vi "WLAN_RSMA_FrameBuild - 2SC.vi"(4 "No. Common Bits":i32=3, 6 "No. Total Bits":i32=6, 7 "Alpha":dbl min=0.0 max=1.0 step=0.05 format="%#_13g", 8 "error in (no error)":errorcluster, 9 "data in 2":i8[](array[numeric]) caption="input bit stream", 10 "Modulation parameter":T1, 11 "data in":i8[](array[numeric]) caption="input bit stream") -> (0 "error out":errorcluster, 3 "output array":cdb[](array[numeric]))   [LabVIEW 2022 SP3]
panel:
  out "Constellation Map":cdb[](graph)
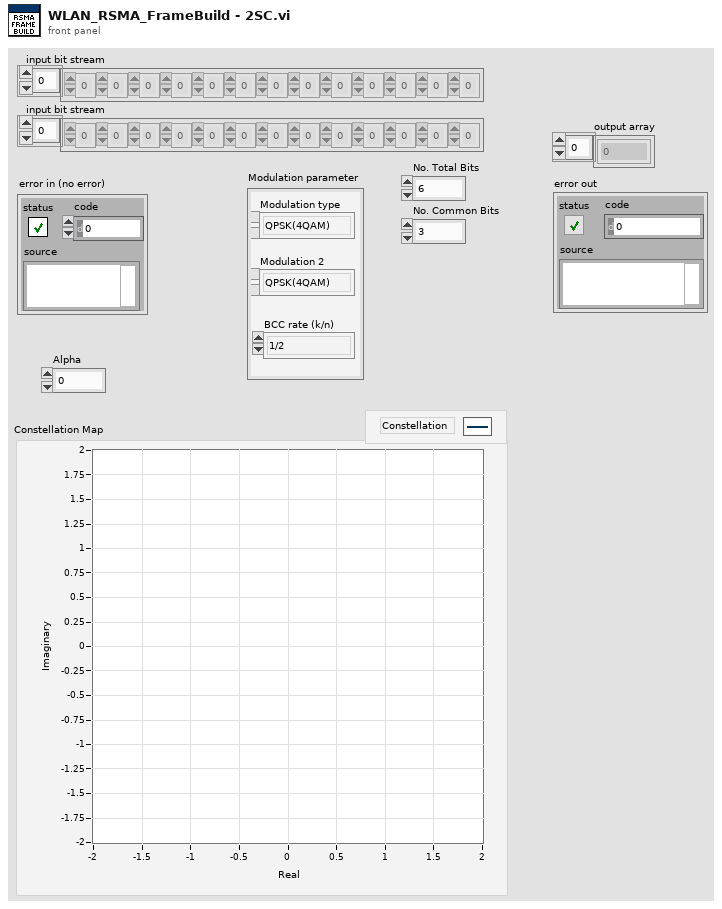
[diagram p1: front panel]
types:
  T1 = cluster{"Modulation type":enum16{"QPSK(4QAM)", "64QAM", "16QAM", "BPSK", "BPSK Vertical"}, "BCC rate (k/n)":enum16{"1/2", "2/3", "3/4"}, "Modulation 2":enum16{"QPSK(4QAM)", "64QAM", "16QAM", "BPSK", "BPSK Vertical"}}
  T2 = enum16{"QPSK(4QAM)", "64QAM", "16QAM", "BPSK", "BPSK Vertical"}
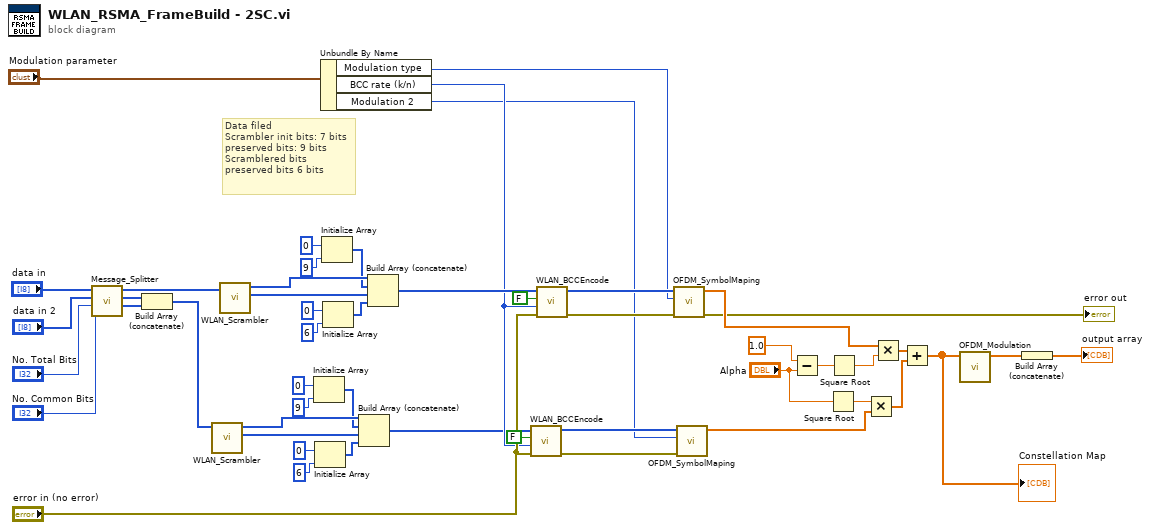
[diagram p0: block diagram]
diagram:
  # "Data filed\nScrambler init bits: 7 bits\npreserved bits: 9 bits\nScramblered bits\npreserved bits 6 bits"
  n1 = call "Message_Splitter.vi"("No. Common Bits"="No. Common Bits", "No. Total Bits"="No. Total Bits", "W2"="data in 2", "W1"="data in") -> ("Wp2"=w9:u8[], "Wp1"=w10:u8[], "Wc"=w8:u8[])  [unwired: 5 in]
  n2 = Build Array (concatenate)(w10, w9) -> (w7:u8[])
  n3 = call "WLAN_Scrambler.vi"("input bit stream"=w7) -> ("scrambled bits"=w27:i8[], "scrambler initial bit"=w31:i8[])  [unwired: 9 in]
  n4 = call "WLAN_Scrambler.vi"("input bit stream"=w8) -> ("scrambled bits"=w23:i8[], "scrambler initial bit"=w38:i8[])  [unwired: 9 in]
  n5 = Initialize Array(i8 0 ("element"), 9 ("dimension size")) -> (w30:i8[])
  n6 = Initialize Array(i8 0 ("element"), 6 ("dimension size")) -> (w24:i8[])
  n7 = Unbundle By Name("Modulation parameter") -> ("Modulation type"=w6:T2, "BCC rate (k/n)"=w46:enum16{"1/2", "2/3", "3/4"}, "Modulation 2"=w3:T2)
  n8 = Initialize Array(i8 0 ("element"), 9 ("dimension size")) -> (w37:i8[])
  n9 = Initialize Array(i8 0 ("element"), 6 ("dimension size")) -> (w32:i8[])
  n10 = Build Array (concatenate)(w31, w30, w27, w24) -> (w43:i8[])
  n11 = Build Array (concatenate)(w38, w37, w23, w32) -> (w50:i8[])
  n12 = call "WLAN_BCCEncode.vi"("error in (no error)"="error in (no error)", "BCC rate (k/n)"=w46, "need add zeros?"=FALSE, "input bit stream"=w43) -> ("error out"=w41:errorcluster, "output bit stream 3"=w42:i8[])  [unwired: 6 in]
  n13 = call "WLAN_BCCEncode.vi"("error in (no error)"="error in (no error)", "BCC rate (k/n)"=w46, "need add zeros?"=FALSE, "input bit stream"=w50) -> ("error out"=w48:errorcluster, "output bit stream 3"=w47:i8[])  [unwired: 6 in]
  n14 = call "OFDM_SymbolMaping.vi"("error in (no error)"=w48, "Modulation type"=w6, "input bit stream"=w47) -> ("error out"=→"error out":errorcluster, "symbols"=w45:cdb[])  [unwired: 7 in]
  n15 = call "OFDM_SymbolMaping.vi"("error in (no error)"=w41, "Modulation type"=w3, "input bit stream"=w42) -> ("symbols"=w40:cdb[])  [unwired: 7 in, 1 out]
  n16 = Subtract(x=1.0, y="Alpha") -> (x-y=w15:dbl)
  n17 = Square Root(x="Alpha") -> (sqrt(x)=w19:dbl)
  n18 = Square Root(x=w15) -> (sqrt(x)=w17:dbl)
  n19 = Multiply(x=w19, y=w40) -> (x*y=w20:cdb[])
  n20 = Multiply(x=w45, y=w17) -> (x*y=w18:cdb[])
  n21 = Add(x=w18, y=w20) -> (x+y=w5:cdb[])
  "Constellation Map" <- w5
  n22 = call "OFDM_Modulation.vi"("Input sequence"=w5) -> ("Output sequence"=w13:cdb[])  [unwired: 10 in]
  n23 = Build Array (concatenate)(w13) -> (→"output array":cdb[])
